vi "xy_weight_height_2.vi"() -> ()   [LabVIEW 2021]
uses:
  <vilib>/Utility/file.llb/Read Delimited Spreadsheet (string).vi
  <vilib>/Analysis/NI_AALBase.lvlib
panel:
  out "Weight Distribution":T1(graph)
  out "Height Distribution":T2(graph)
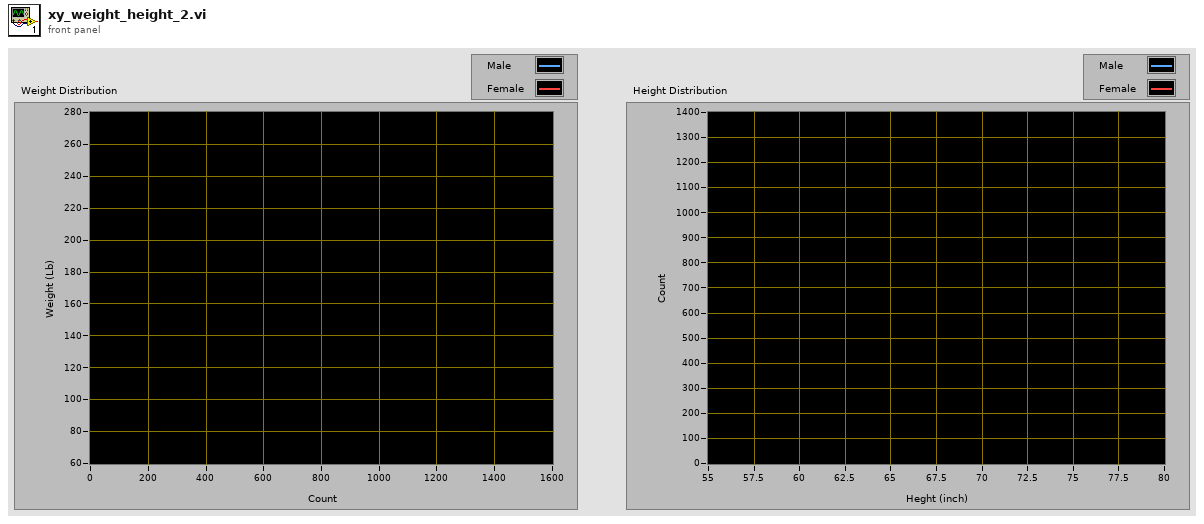
[diagram p1: front panel]
types:
  T1 = cluster{"Histogram: h(x)":i32[], "X Values":dbl[]}[]
  T2 = cluster{"X Values":dbl[], "Histogram: h(x)":i32[]}[]
  T3 = cluster{"X Values":dbl[], "Histogram: h(x)":i32[]}
  T4 = cluster{"Histogram: h(x)":i32[], "X Values":dbl[]}
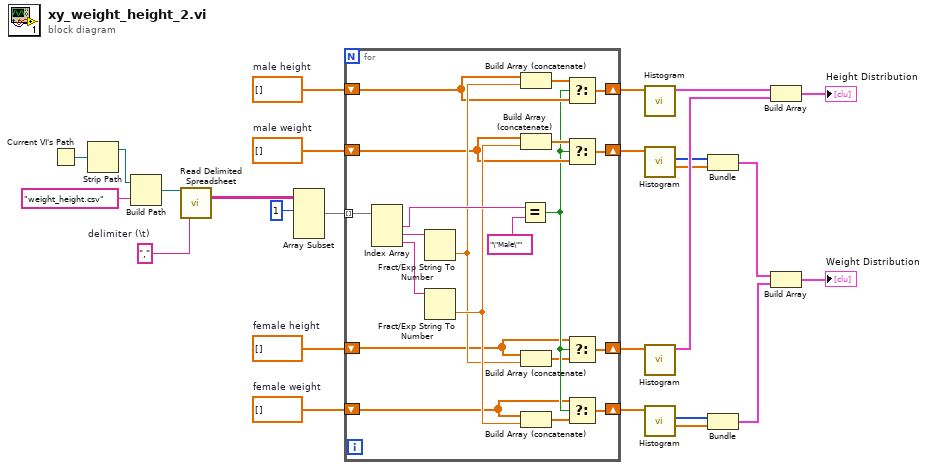
[diagram p0: block diagram]
diagram:
  w15 = dbl[] []  # female weight
  w16 = dbl[] []  # female height
  w17 = dbl[] []  # male weight
  w18 = dbl[] []  # male height
  w22 = ","  # delimiter (\t)
  n1 = Current VI's Path() -> (path=w26:path)
  n2 = Strip Path(path=w26) -> (stripped path=w25:path)  [unwired: 1 out]
  n3 = Build Path(base path=w25, name or relative path="weight_height.csv") -> (appended path=w23:path)
  n4 = call-poly <vilib>:"Read Delimited Spreadsheet.vi"("file path (dialog if empty)"=w23, "delimiter (\\t)"=w22) -> ("all rows"=w21:string[][])  [unwired: 8 in, 5 out]
  n5 = Array Subset(array=w21, index (row)=1 ("index")) -> (w19:string[][])  [unwired: 3 in]
  n6 = for {
    tunnel: w19 -> [w46] mode=indexing
    shift-right: [w41] -> w14
    shift-left: w18 -> [w35]
    shift-right: [w38] -> w13
    shift-left: w17 -> [w34]
    shift-right: [w27] -> w12
    shift-left: w16 -> [w32]
    shift-right: [w28] -> w11
    shift-left: w15 -> [w31]
    n7 = Index Array(array=w46) -> (element #1=w45:string, element #2=w43:string, element #3=w39:string)  [unwired: 3 in]
    n8 = Fract/Exp String To Number(string=w43) -> (number=w36:dbl)  [unwired: 3 in, 1 out]
    n9 = Fract/Exp String To Number(string=w39) -> (number=w37:dbl)  [unwired: 3 in, 1 out]
    n10 = Equal?(x=w45, y="\"Male\"") -> (x = y?=w33:bool)
    n11 = Build Array (concatenate)(w35, w36) -> (w42:dbl[])
    n12 = Build Array (concatenate)(w34, w37) -> (w40:dbl[])
    n13 = Build Array (concatenate)(w32, w36) -> (w30:dbl[])
    n14 = Build Array (concatenate)(w31, w37) -> (w29:dbl[])
    n15 = Select(t=w42, s=w33, f=w35) -> (s? t:f=w41:dbl[])
    n16 = Select(t=w40, s=w33, f=w34) -> (s? t:f=w38:dbl[])
    n17 = Select(t=w32, s=w33, f=w30) -> (s? t:f=w27:dbl[])
    n18 = Select(t=w31, s=w33, f=w29) -> (s? t:f=w28:dbl[])
  }
  n19 = call <vilib>:"Histogram.vi"("X"=w14) -> ("Histogram Graph"=w10:T3)  [unwired: 7 in, 3 out]
  n20 = call <vilib>:"Histogram.vi"("X"=w13) -> ("X Values"=w3:dbl[], "Histogram: h(x)"=w4:i32[])  [unwired: 7 in, 2 out]
  n21 = call <vilib>:"Histogram.vi"("X"=w12) -> ("Histogram Graph"=w9:T3)  [unwired: 7 in, 3 out]
  n22 = call <vilib>:"Histogram.vi"("X"=w11) -> ("X Values"=w1:dbl[], "Histogram: h(x)"=w2:i32[])  [unwired: 7 in, 2 out]
  n23 = Bundle("Histogram: h(x)"=w4, "X Values"=w3) -> (w7:T4)  [unwired: 1 in]
  n24 = Bundle("Histogram: h(x)"=w2, "X Values"=w1) -> (w6:T4)  [unwired: 1 in]
  n25 = Build Array(w10, w9) -> (→"Height Distribution":T2)
  n26 = Build Array(w7, w6) -> (→"Weight Distribution":T1)
